vi "PurgeAsH3_00.vi"() -> ()   [LabVIEW 2011]
uses:
  <vilib>/Platform/TimedLoop/XDataNode/timing_clust.ctl
  <vilib>/Platform/TimedLoop/XDataNode/nitl_modes.ctl
  <vilib>/Platform/TimedLoop/XDataNode/wakeup.ctl
  <vilib>/Platform/TimedLoop/XDataNode/XDataNode.xnode
  <vilib>/Platform/TimedLoop/XDataNode/XDNodeRunTimeDep.lvlib
panel:
  in  "Numeric 3":dbl caption="fill wait (s)"
  in  "Numeric 2":dbl caption="evacuation wait (s)"
  out "As Gas Actual Flow Rate 2":dbl caption="evacuation flow"
  out "As Gas Actual Flow Rate":dbl caption="fill flow"
  out "Numeric":i32 caption="iteration"
  in  "y2":dbl=95.0 caption="fill threshold"
  in  "y":dbl=5.0 caption="evacuation threshold"
  in  "Iterations":i32=20
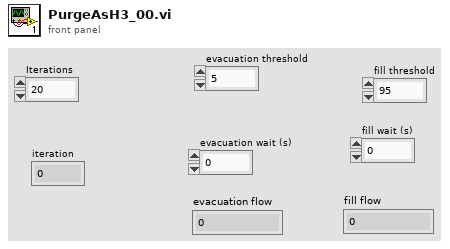
[diagram p1: front panel]
types:
  T1 = typedef "XDNodeRunTimeDep.lvlib/timing_clust.ctl" = cluster{"Expected End [f-1]":u64, "Actual End [f-1]":u64, "Finished Late? [f-1]":bool, "Expected End [i-1]":u64, "Actual End [i-1]":u64, "Finished Late? [i-1]":bool, "Expected Start [i]":u64, "Actual Start [i]":u64, "Expected Start [f]":u64, "Actual Start [f]":u64, "Source Name":string, "Structure Name":string, "Period":i64, "Deadline":i64, "Offset":i64, "Start":i64, "Priority":i32, "Timeout":i32, "Mode":T2, "Wakeup Reason":T3, "Error":errorcluster, "Source Type":string, "Secondary Source Type":string, "Global End Time":u64, "Global Start Time":u64, "Frame Duration":u64, "Iteration Duration":u64, "Assigned CPU":i32, "I/O Scan Engine Mode":u32}
  T2 = typedef "XDNodeRunTimeDep.lvlib/nitl_modes.ctl" = enum32{"No Change", "Process missed periods, maintain original phase", "Discard missed periods, maintain original phase", "Process missed periods, ignore original phase", "Discard missed periods, ignore original phase"}
  T3 = typedef "XDNodeRunTimeDep.lvlib/wakeup.ctl" = enum32{"Normal", "Aborted", "Asynchronous wakeup", "Timing source error", "Timed loop error", "Timeout"}
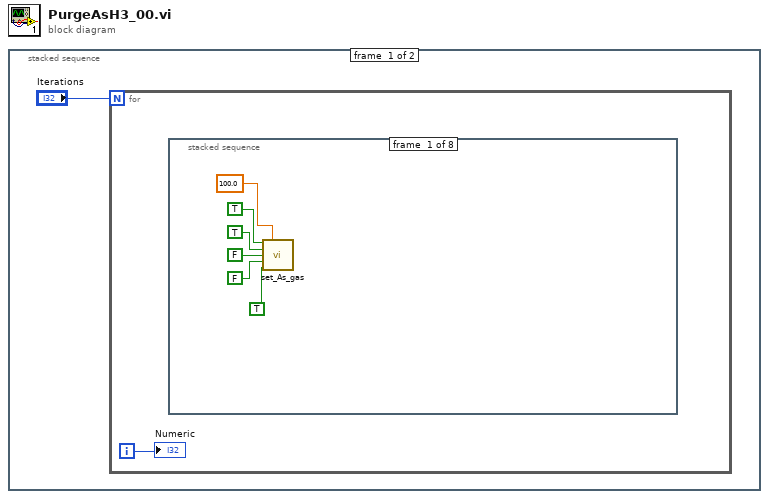
[diagram p0: block diagram]
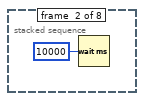
[diagram p2: hidden frame]
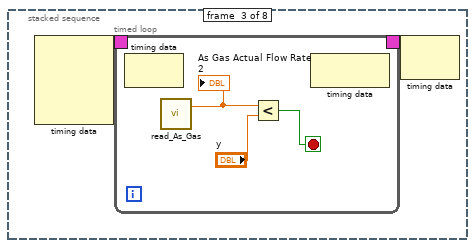
[diagram p3: hidden frame]
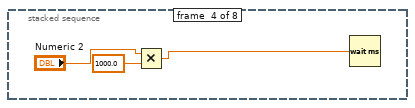
[diagram p4: hidden frame]
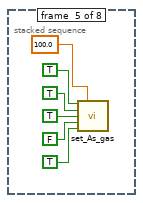
[diagram p5: hidden frame]
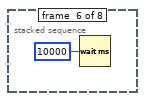
[diagram p6: hidden frame]
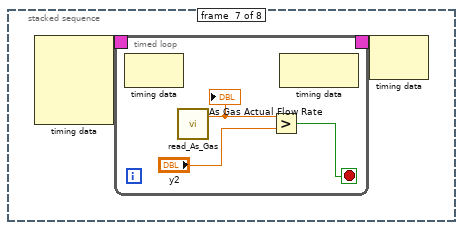
[diagram p7: hidden frame]
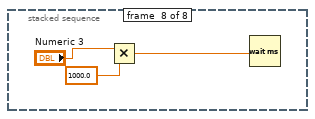
[diagram p8: hidden frame]
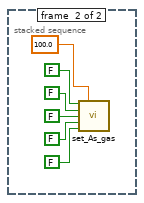
[diagram p9: hidden frame]
diagram:
  n1 = stacked-sequence {
    frame #0 {
      n2 = for {
        N: "Iterations" -> [_]
        i -> [w2]
        n3 = stacked-sequence {
          frame #0 {
            n4 = call "set_As_gas.vi"("As_Gas Active"=TRUE, "As_Gas Flow"=100.0, "As_Gas In"=TRUE, "As_Gas H2"=FALSE, "As_Gas Run"=FALSE, "As_Gas Remote"=TRUE) -> ()  [unwired: 10 in]
          }
          frame #1 {
            n5 = Wait (ms)(milliseconds to wait=u32 10000) -> ()  [unwired: 1 out]
          }
          frame #2 {
            n6 = node-c288() -> (w11:T1)  [unwired: 4 in]
            n7 = timed-loop {
              timing: w11 -> [_]
              timing-out: [_] -> w10
              stop <- w12 stop-if-true
              n8 = node-c288() -> ()  [unwired: 1 in, 1 out]
              n9 = call "read_As_Gas.vi"() -> ("As Gas Actual Flow Rate"=w14:dbl)  [unwired: 5 out]
              "As Gas Actual Flow Rate 2" <- w14
              n10 = Less?(x=w14, y="y") -> (x < y?=w12:bool)
              n11 = node-c288() -> ()  [unwired: 1 in, 1 out]
            }
            n12 = node-c288(w10) -> ()  [unwired: 1 out]
          }
          frame #3 {
            n13 = Multiply(x="Numeric 2", y=1000.0) -> (x*y=w19:dbl)
            n14 = Wait (ms)(milliseconds to wait=w19) -> ()  [unwired: 1 out]
          }
          frame #4 {
            n15 = call "set_As_gas.vi"("As_Gas Active"=TRUE, "As_Gas Flow"=100.0, "As_Gas In"=TRUE, "As_Gas H2"=TRUE, "As_Gas Run"=FALSE, "As_Gas Remote"=TRUE) -> ()  [unwired: 10 in]
          }
          frame #5 {
            n16 = Wait (ms)(milliseconds to wait=u32 10000) -> ()  [unwired: 1 out]
          }
          frame #6 {
            n17 = node-c288() -> (w30:T1)  [unwired: 4 in]
            n18 = timed-loop {
              timing: w30 -> [_]
              timing-out: [_] -> w29
              stop <- w31 stop-if-true
              n19 = node-c288() -> ()  [unwired: 1 in, 1 out]
              n20 = call "read_As_Gas.vi"() -> ("As Gas Actual Flow Rate"=w33:dbl)  [unwired: 5 out]
              "As Gas Actual Flow Rate" <- w33
              n21 = Greater?(x=w33, y="y2") -> (0:w31:bool)
              n22 = node-c288() -> ()  [unwired: 1 in, 1 out]
            }
            n23 = node-c288(w29) -> ()  [unwired: 1 out]
          }
          frame #7 {
            n24 = Multiply(x="Numeric 3", y=1000.0) -> (x*y=w38:dbl)
            n25 = Wait (ms)(milliseconds to wait=w38) -> ()  [unwired: 1 out]
          }
        }
        "Numeric" <- w2
      }
    }
    frame #1 {
      n26 = call "set_As_gas.vi"("As_Gas Active"=FALSE, "As_Gas Flow"=100.0, "As_Gas In"=FALSE, "As_Gas H2"=FALSE, "As_Gas Run"=FALSE, "As_Gas Remote"=FALSE) -> ()  [unwired: 10 in]
    }
  }
